vi "GetFromAPI.vi"(8 "error in (no error)":errorcluster, 11 "ClashRoyale in":refnum<class "StashRoyale.lvclass">) -> (0 "error out":errorcluster, 2 "JSON response":string, 3 "ClashRoyale out":refnum<class "StashRoyale.lvclass">)   [LabVIEW 2020, in "StashRoyale.lvclass"]
uses:
  StashRoyale.lvclass
  <vilib>/addons/Tools/Unicode/UTF8 Tools.lvlib
  support/JSON.lvlibp
  ctl_ClientError.ctl
panel:
  in  "Argument":string
  in  "API GET":T1(ring)
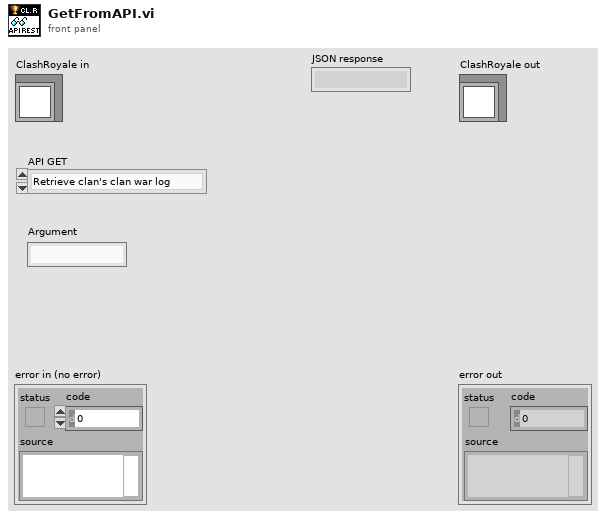
[diagram p1: front panel]
types:
  T1 = enum16{"Retrieve clan's clan war log", "Search clans", "Retrieve clan's river race log", "Retrieve information about clan's current clan war", "Get clan information", "List clan members", "Retrieve information about clan's current river race", "Get player information", "Get information about player's upcoming chests", "Get list of recent battles for a player", "Get list of available cards", "Search tournaments", "Get tournament information", "Get clan rankings for a specific location", "Get player rankings for a specific location", "Get clan war rankings for a specific location", "Get top Path of Legend players for given season", "Get top player league season", "Get top player rankings for a season", "Lists top player league seasons.", "List locations", "Get location information", "Get current and upcoming challenges", "Get list of global tournaments"}
  T2 = typedef "StashRoyale.lvclass/ctl_ErrorCodes.ctl" = i32
  T3 = typedef "StashRoyale.lvclass/ctl_ClientError.ctl" = cluster{"reason":string, "message":string, "type":string}
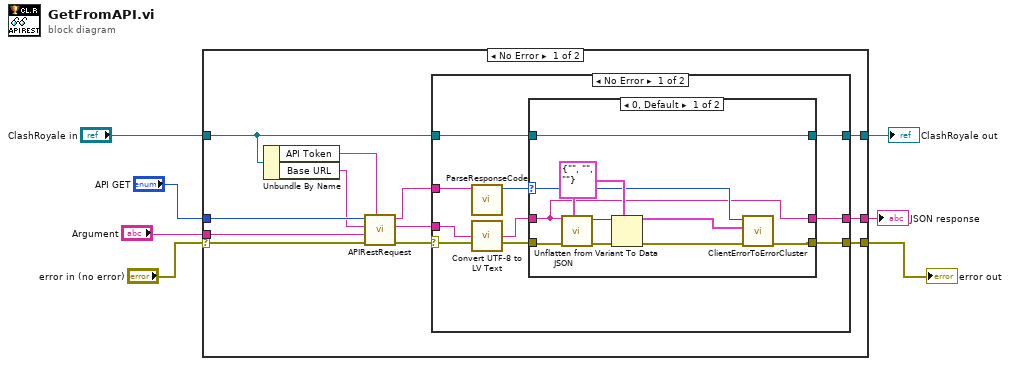
[diagram p0: block diagram]
diagram:
  n1 = case shown="No Error" "error in (no error)" {
    selector: "error in (no error)" -> [w18 w46]
    tunnel: [w14 w46] -> w6
    tunnel: [w16 w45] -> w4
    tunnel: "ClashRoyale in" -> [w17 w45]
    tunnel: [w12 _] -> w3
    tunnel: "API GET" -> [w11 _]
    tunnel: "Argument" -> [w8 _]
    frame No Error {
      n2 = Unbundle By Name(w17) -> ("API Token"=w9:string, "Base URL"=w10:string)
      n3 = call "APIRestRequest.vi"("API Token"=w9, "error in (no error)"=w18, "Argument"=w8, "Base URL"=w10, "API GET"=w11) -> ("error out"=w15:errorcluster, "body"=w19:string, "headers"=w13:string)  [unwired: 4 in]
      n4 = case shown="No Error" w15 {
        selector: w15 -> [w26 w43]
        tunnel: w19 -> [w29 _]
        tunnel: w17 -> [w28 w44]
        tunnel: [w27 w44] -> w16
        tunnel: [w23 w43] -> w14
        tunnel: w13 -> [w22 _]
        tunnel: [w20 _] -> w12
        frame No Error {
          n5 = call "ParseResponseCode.vi"("Response Header"=w22) -> ("response code (200)"=w21:T2)  [unwired: 10 in]
          n6 = call <vilib>:"Convert UTF-8 to LV Text.vi"("UTF-8 Text"=w29, "error in"=w26) -> ("LV Text"=w25:string, "error out"=w24:errorcluster)  [unwired: 12 in]
          n7 = case shown="0, Default" w21 {
            selector: w21 -> [w32 _]
            tunnel: w28 -> [w39 w41]
            tunnel: [w39 w41] -> w27
            tunnel: w25 -> [w30 w40]
            tunnel: w24 -> [w36 w42]
            tunnel: [w31 w42] -> w23
            tunnel: [w30 w40] -> w20
            frame 0, Default {
              w35 = T3 {"reason"="", "message"="", "type"=""} ("ClientError")
              n8 = call "Unflatten from JSON.vi"("Type and Defaults"=w35, "error in (no error)"=w36, "JSON String"=w30) -> ("error out"=w37:errorcluster, "data"=w38:variant)  [unwired: 7 in]
              n9 = Variant To Data(error in=w37, type=w35, Variant=w38) -> (data=w33:T3, error out=w34:errorcluster)
              n10 = call "ClientErrorToErrorCluster.vi"("error in (no error)"=w34, "ClientError"=w33, "response code (200)"=w32) -> ("error out"=w31:errorcluster)  [unwired: 8 in]
            }
            frame 200 {
            }
          }
        }
        frame Error {
        }
      }
    }
    frame Error {
    }
  }
  "error out" <- w6
  "ClashRoyale out" <- w4
  "JSON response" <- w3
